vi "get_config_cluster.vi"(8 "error in (no error)":errorcluster, 11 "GenericPlugin in":refnum<class "DAQ_MG090622Camera.lvclass">) -> (0 "error out":errorcluster, 2 "config cluster (variant)":variant, 3 "GenericPlugin out":refnum<class "DAQ_MG090622Camera.lvclass">)   [LabVIEW 2010, in "DAQ_MG090622Camera.lvclass"]
uses:
  DAQ_MG090622Camera.lvclass
  DAQ_MG090622Camera.lvclass/DAQ_MG090622Camera.ctl
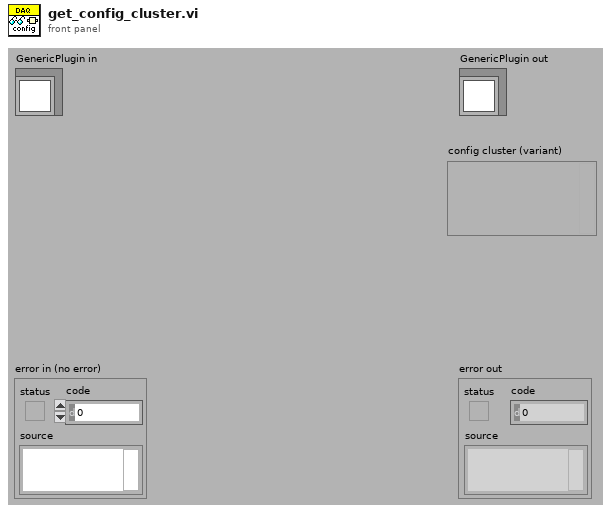
[diagram p1: front panel]
types:
  T1 = typedef "DAQ_MG090622Camera.lvclass/config_data_cluster.ctl" = cluster{"device name":string, "camera type":T2, "connection type":T3}
  T2 = typedef "DAQ_MG090622Camera.lvclass/camera_type_enum.ctl" = enum16{"gray scale", "RGB"}
  T3 = typedef "DAQ_MG090622Camera.lvclass/connection_type_enum.ctl" = enum16{"IEEE 1394 (FireWire)", "USB", "GigE", "CameraLink"}
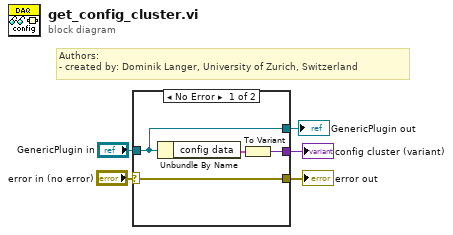
[diagram p0: block diagram]
diagram:
  # "Authors: \n- created by: Dominik Langer, University of Zurich, Switzerland"
  n1 = case shown="No Error" "error in (no error)" {
    selector: "error in (no error)" -> [w7 w11]
    tunnel: "GenericPlugin in" -> [w6 w10]
    tunnel: [w8 _] -> w4
    tunnel: [w7 w11] -> w2
    tunnel: [w6 w10] -> w1
    frame No Error {
      n2 = Unbundle By Name(w6) -> ("config data"=w9:T1)
      n3 = To Variant(anything=w9) -> (Variant=w8:variant)
    }
    frame Error {
    }
  }
  "error out" <- w2
  "GenericPlugin out" <- w1
  "config cluster (variant)" <- w4
